vi "ReduceVariables.vi"(1 "Script in":string) -> (0 "Script out":string)   [LabVIEW 2012]
panel:
  out "reduction":bool[](array[boolean])
  out "# occ":i32[](array[numeric])
  out "variable":string[](array[string])
  out "Array":string[](array[string])
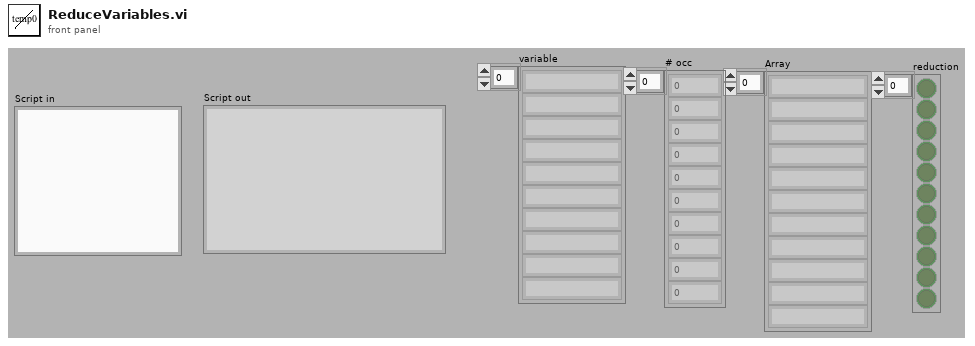
[diagram p1: front panel]
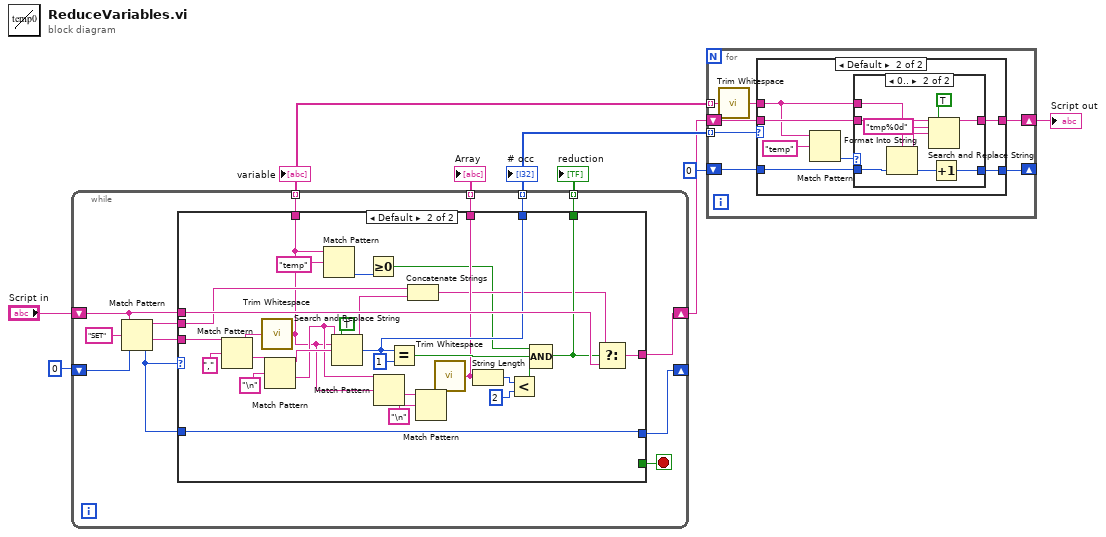
[diagram p0: block diagram]
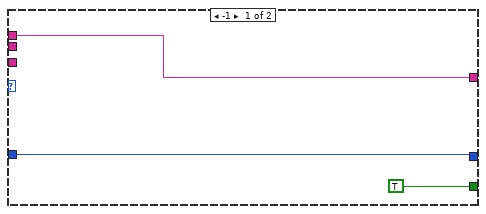
[diagram p4: hidden frame]
diagram:
  n1 = while {
    shift-right: [w16] -> w2
    shift-left: "Script in" -> [w20]
    shift-right: [w15] -> _
    shift-left: 0 ("y") -> [w18]
    tunnel: [w14] -> w7 mode=indexing
    tunnel: [w12] -> w5 mode=indexing
    tunnel: [w11] -> w4 mode=indexing
    tunnel: [w10] -> w6 mode=indexing
    stop <- w17 stop-if-true
    n2 = Match Pattern(string=w20, regular expression="SET", offset (0)=w18) -> (before substring=w19:string, after substring=w21:string, offset past match=w13:i32)  [unwired: 1 out]
    n3 = case shown="Default" w13 {
      tunnel: w21 -> [_ w29]
      tunnel: w20 -> [w25 w48]
      tunnel: [w25 w39] -> w16
      tunnel: w19 -> [_ w34]
      tunnel: w13 -> [w24 w30]
      tunnel: [w24 w30] -> w15
      tunnel: [TRUE _] -> w17
      tunnel: [_ w36] -> w14
      tunnel: [_ w28] -> w12
      tunnel: [_ w37] -> w11
      tunnel: [_ w35] -> w10
      frame -1 {
      }
      frame Default {
        n4 = Match Pattern(string=w29, regular expression=",") -> (before substring=w43:string, after substring=w52:string)  [unwired: 1 in, 2 out]
        n5 = call <vilib>:"Trim Whitespace.vi"("string"=w43) -> ("trimmed string"=w28:string)  [unwired: 1 in]
        n6 = Match Pattern(string=w52, regular expression="\n") -> (before substring=w50:string, after substring=w38:string)  [unwired: 1 in, 2 out]
        n7 = Match Pattern(string=w28, regular expression="temp") -> (offset past match=w26:i32)  [unwired: 1 in, 3 out]
        n8 = Search and Replace String(replace all?=TRUE ("replace all? (F)"), input string=w38, search string=w28, replace string=w50) -> (result string=w33:string, number of replacements=w37:i32)  [unwired: 4 in, 2 out]
        n9 = Greater Or Equal To 0?(x=w26) -> (x >= 0?=w31:bool)
        n10 = Match Pattern(string=w38, regular expression=w28) -> (after substring=w42:string)  [unwired: 1 in, 3 out]
        n11 = Equal?(x=w37, y=1) -> (x = y?=w47:bool)
        n12 = Concatenate Strings(w34, w33) -> (w32:string)
        n13 = Match Pattern(string=w42, regular expression="\n") -> (before substring=w41:string)  [unwired: 1 in, 3 out]
        n14 = call <vilib>:"Trim Whitespace.vi"("string"=w41) -> ("trimmed string"=w36:string)  [unwired: 1 in]
        n15 = String Length(string=w36) -> (length=w40:i32)
        n16 = Less?(x=w40, y=2) -> (x < y?=w44:bool)
        n17 = Compound Arithmetic op=AND(w31, w47, w44) -> (w35:bool)
        n18 = Select(t=w32, s=w35, f=w48) -> (s? t:f=w39:string)
      }
    }
  }
  "Array" <- w7
  "variable" <- w5
  "# occ" <- w4
  "reduction" <- w6
  n19 = for {
    tunnel: w5 -> [w58] mode=indexing
    tunnel: w4 -> [w61] mode=indexing
    shift-right: [w56] -> _
    shift-left: 0 ("y") -> [w57]
    shift-right: [w59] -> w1
    shift-left: w2 -> [w60]
    n20 = call <vilib>:"Trim Whitespace.vi"("string"=w58) -> ("trimmed string"=w55:string)  [unwired: 1 in]
    n21 = case shown="Default" w61 {
      tunnel: w60 -> [w63 w70]
      tunnel: [w63 w69] -> w59
      tunnel: w55 -> [_ w66]
      tunnel: w57 -> [w62 w68]
      tunnel: [w62 w67] -> w56
      frame 0, 1 {
      }
      frame Default {
        n22 = Match Pattern(string=w66, regular expression="temp") -> (offset past match=w64:i32)  [unwired: 1 in, 3 out]
        n23 = case shown="0.." w64 {
          tunnel: w70 -> [w72 w79]
          tunnel: [w72 w78] -> w69
          tunnel: w68 -> [w71 w76]
          tunnel: [w71 w75] -> w67
          tunnel: w66 -> [_ w73]
          frame Default {
          }
          frame 0.. {
            n24 = Format Into String(format string="tmp%0d", w76) -> (resulting string=w74:string)  [unwired: 2 in, 1 out]
            n25 = Search and Replace String(replace all?=TRUE ("replace all? (F)"), input string=w79, search string=w73, replace string=w74) -> (result string=w78:string)  [unwired: 4 in, 3 out]
            n26 = Increment(x=w76) -> (x+1=w75:i32)
          }
        }
      }
    }
  }
  "Script out" <- w1
